vi "Main.vi"(8 "error in":errorcluster, 11 "Check all Worker Queues in":refnum<class "_Check all Worker Queues.lvclass">) -> (0 "error out":errorcluster, 3 "Check all Worker Queues out":refnum<class "_Check all Worker Queues.lvclass">)   [LabVIEW 2017, in "_Check all Worker Queues.lvclass"]
doc: "The <b>Queued Message Handler</b> of the Worker that owns this VI."
uses:
  _Check all Worker Queues.lvclass
  C:/Program Files (x86)/National Instruments/LabVIEW 2017/vi.lib/addons/_Workers/Library/Classes/Worker/Worker.lvclass
  Initialization Data.ctl
  Response Cases.ctl
  <vilib>/addons/_Workers/Library/Case Label.ctl
  _Check all Worker Queues.lvclass/_Check all Worker Queues.ctl
  rwr_Get Number of Elements in all Queues.ctl
  rwr_Get Number of Elements in all Queues Reply.ctl
  <vilib>/addons/_Workers/Library/Classes/Message Queue/Message Queue.lvclass
  <vilib>/addons/_Workers/Library/Workers.lvlib
panel:
  out "Multicolumn Listbox":i32(listbox)
  in  "Check Queues":bool
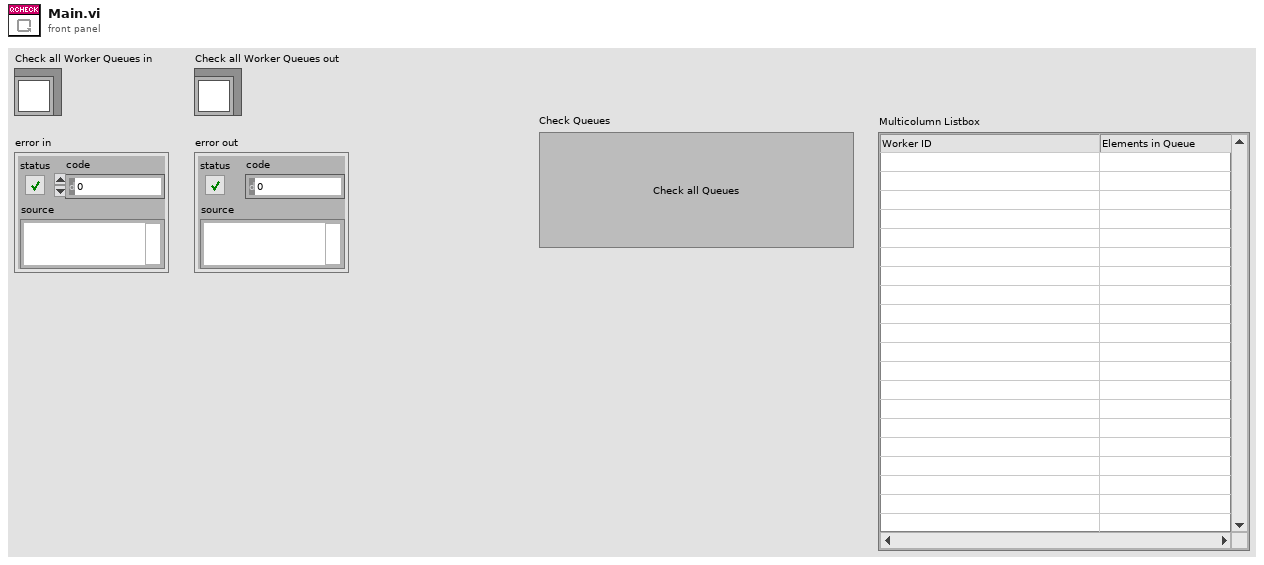
[diagram p1: front panel]
types:
  T1 = typedef "_Check all Worker Queues.lvclass/Initialization Data.ctl" = cluster{"Response Cases":T2}
  T2 = typedef "_Check all Worker Queues.lvclass/Response Cases.ctl" = cluster{"Placeholder - Can be deleted":string, "Get Number of Elements in all Queues_":T3}
  T3 = typedef "Workers.lvlib/Case Label.ctl" = string
  T4 = typedef "_Check all Worker Queues.lvclass/rwr_Get Number of Elements in all Queues Reply.ctl" = cluster{"Elements in Queues":string[][]}
  T5 = typedef "_Check all Worker Queues.lvclass/rwr_Get Number of Elements in all Queues.ctl" = cluster{"String":string}
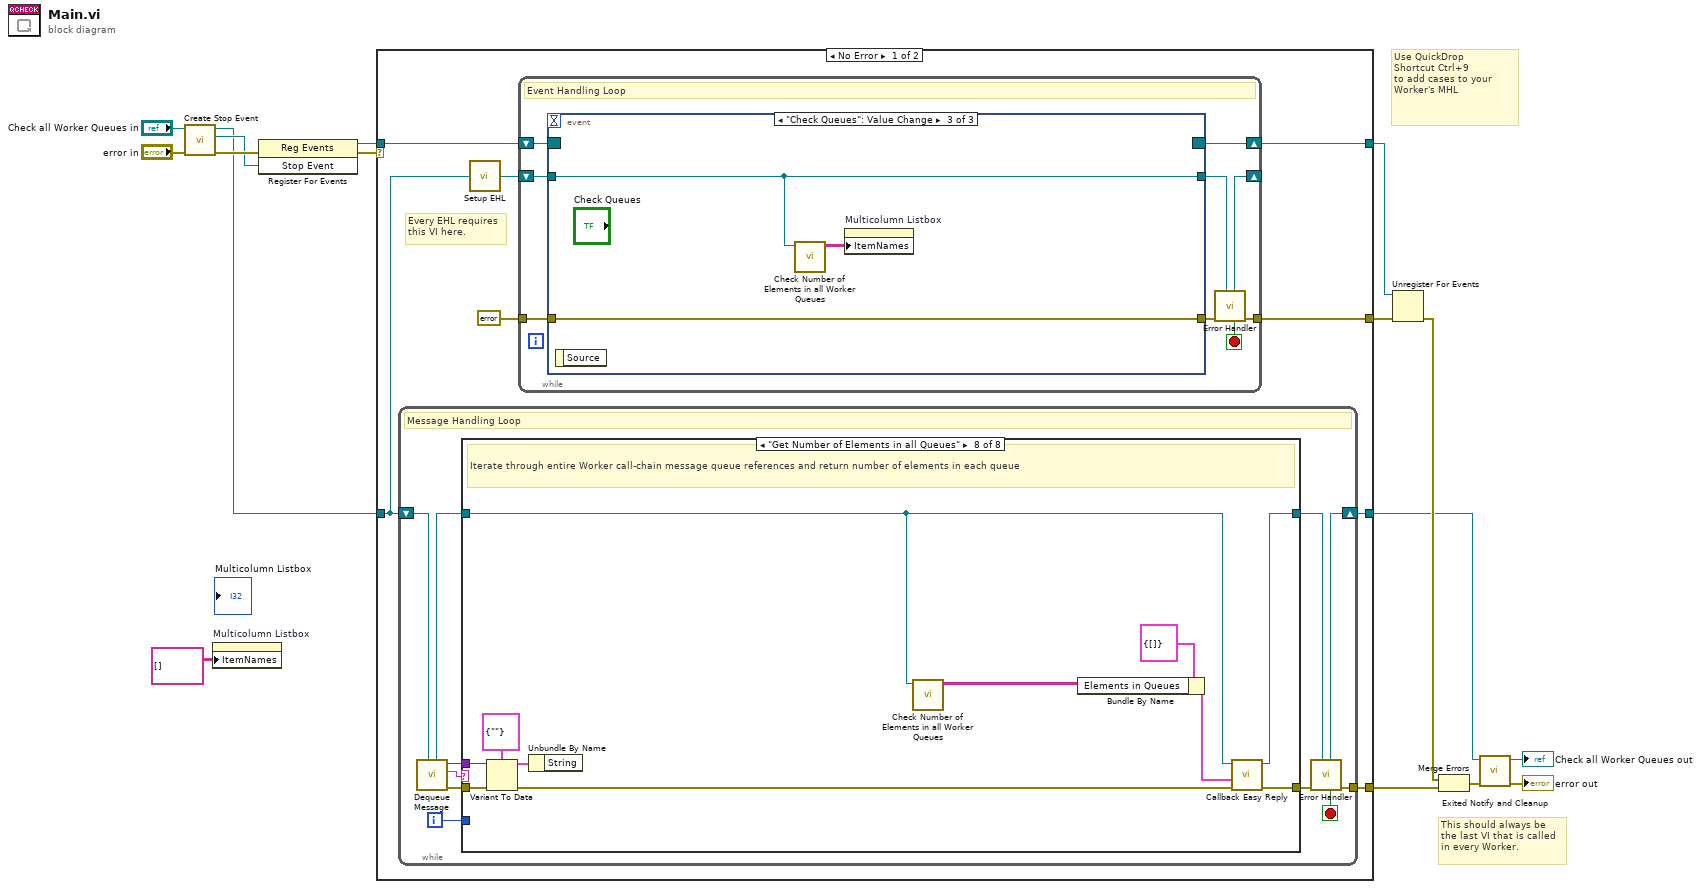
[diagram p0: block diagram]
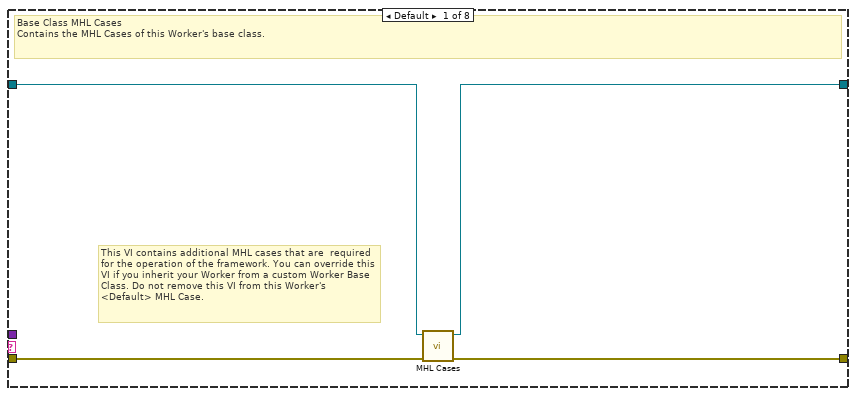
[diagram p2: hidden frame]
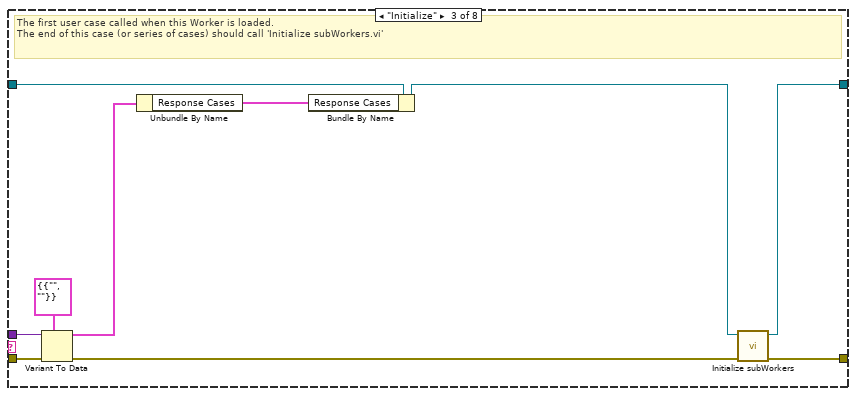
[diagram p4: hidden frame]
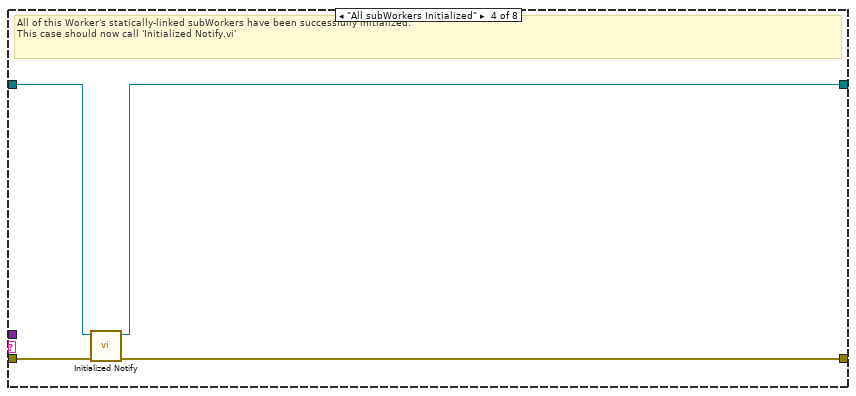
[diagram p5: hidden frame]
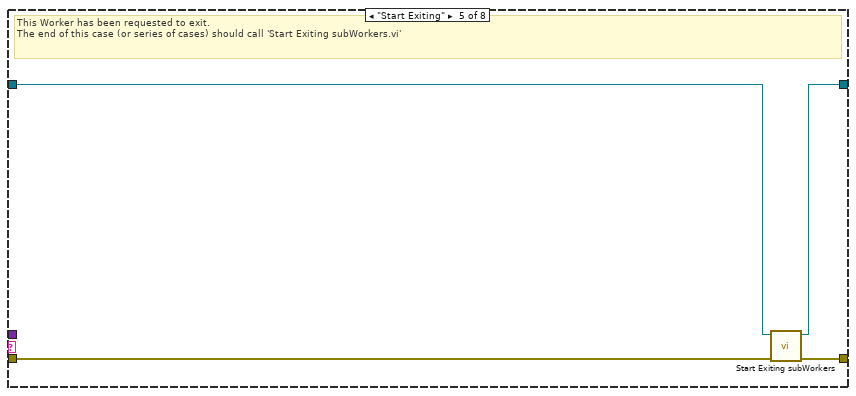
[diagram p6: hidden frame]
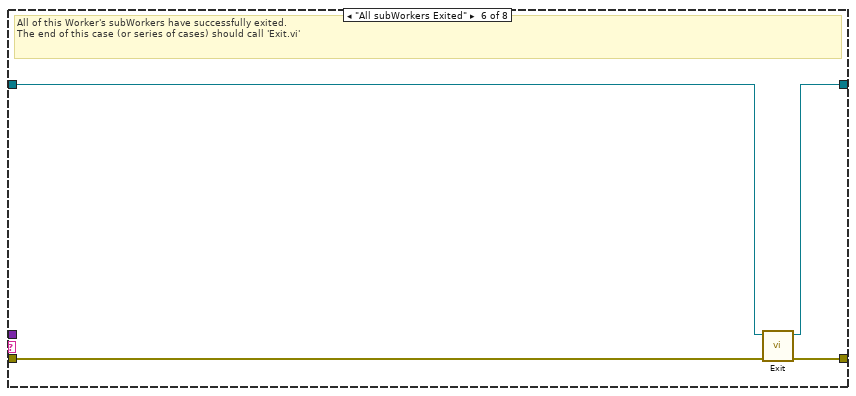
[diagram p7: hidden frame]
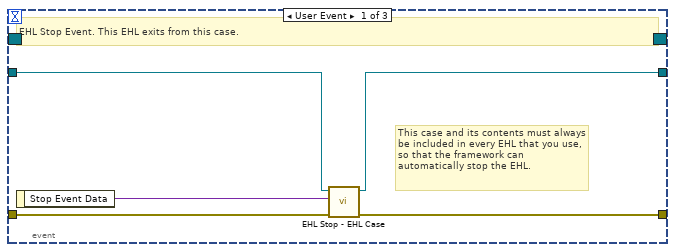
[diagram p9: hidden frame]
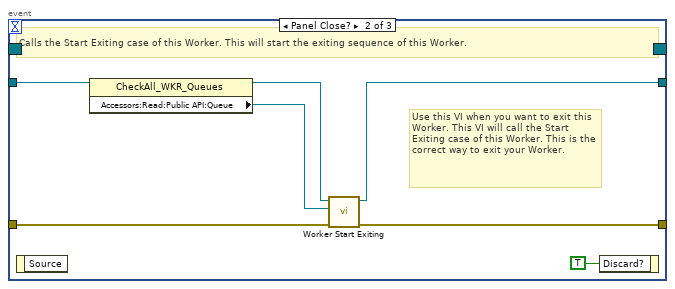
[diagram p10: hidden frame]
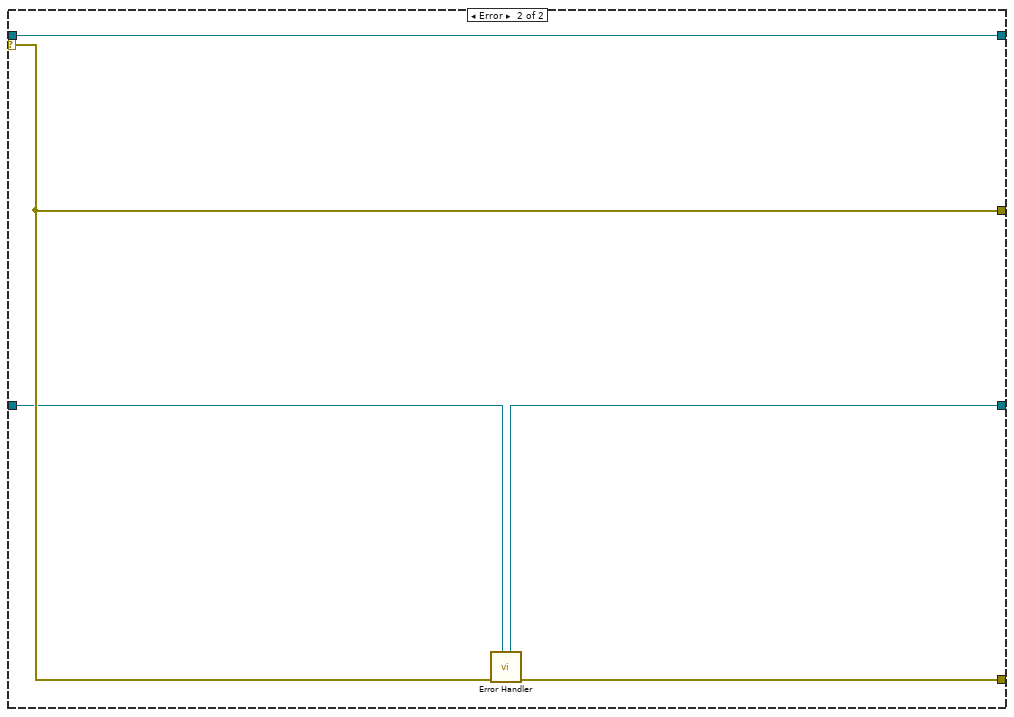
[diagram p11: hidden frame]
diagram:
  # "Use QuickDrop\nShortcut Ctrl+9\nto add cases to your\nWorker's MHL"
  # "This should always be the last VI that is called in every Worker."
  n1 = call-dynamic "Create Stop Event.vi"("error in"="error in", "Worker"="Check all Worker Queues in") -> ("error out"=w11:errorcluster, "Stop Event"=w8:refnum<user-event>, "Worker out"=w5:refnum<class "_Check all Worker Queues.lvclass">)  [unwired: 7 in]
  n2 = property on="Multicolumn Listbox" class="MCListbox (strict)"("ItemNames"=string[][] [] ("Item Names")) -> ()  [unwired: 2 in, 2 out]
  n3 = register-events(error in=w11, w8) -> (reference out=w10:refnum<event-registration>, error out=w2:errorcluster)  [unwired: 1 in]
  n4 = case shown="No Error" w2 {
    tunnel: w5 -> [w19 w102]
    tunnel: [w17 w103] -> w9
    tunnel: w10 -> [w24 w104]
    tunnel: [w21 w105] -> w15
    tunnel: [w23 w104] -> w14
    tunnel: [w18 w101] -> w12
    selector: w2 -> [_ w105]
    frame No Error {
      # "Every EHL requires\nthis VI here."
      n5 = while {
        shift-right: [w33] -> w18
        shift-left: w19 -> [w35]
        tunnel: [w34] -> w17
        i -> [w26]
        stop <- w27 stop-if-true
        # "Message Handling Loop"
        n6 = call-dynamic "Dequeue Message.vi"("Worker"=w35) -> ("error out"=w32:errorcluster, "Case out"=w28:string, "Data out"=w25:variant, "Worker out"=w30:refnum<class "_Check all Worker Queues.lvclass">)  [unwired: 6 in, 1 out]
        n7 = case "Worker MHL Case Structure (DO NOT CHANGE LABEL NAME)" shown="\"Get Number of Elements in all Queues\"" w28 {
          tunnel: w32 -> [w39 w40 w49 w53 w56 w63 w65 w76]
          tunnel: [w38 w40 w51 w52 w59 w62 w65 w71] -> w31
          tunnel: w30 -> [w37 w41 w48 w55 w57 w61 w64 w68]
          tunnel: [w36 w41 w50 w54 w58 w60 w64 w70] -> w29
          tunnel: w26 -> [_ _ _ _ _ _ _ _]
          tunnel: w25 -> [_ _ w46 _ _ _ _ w73]
          frame Default {
            # "This VI contains additional MHL cases that are  required for the operation of the framework. You can override this VI if you inherit your Worker from a custom Worker Base Class. Do not remove this VI from this Worker's <Default> MHL Case."
            # "Base Class MHL Cases\nContains the MHL Cases of this Worker's base class."
            n8 = call-dynamic "MHL Cases.vi"("error in"=w39, "Worker in"=w37) -> ("error out"=w38:errorcluster, "Worker out"=w36:refnum<class "_Check all Worker Queues.lvclass">)  [unwired: 8 in]
          }
          frame "------------ FRAMEWORK CASES -----------" {
            # "Start of Workers Framework Cases"
          }
          frame "Initialize" {
            # "The first user case called when this Worker is loaded.\nThe end of this case (or series of cases) should call 'Initialize subWorkers.vi'"
            n9 = Variant To Data(error in=w49, type=T1 {"Response Cases"={"Placeholder - Can be deleted"="", "Get Number of Elements in all Queues_"=""}} ("Initialization Data"), Variant=w46) -> (data=w44:T1, error out=w47:errorcluster)
            n10 = Unbundle By Name(w44) -> ("Response Cases"=w43:T2)
            n11 = Bundle By Name(cluster=w48, "Response Cases"=w43) -> (w45:refnum<class "_Check all Worker Queues.lvclass">)
            n12 = call-dynamic "Initialize subWorkers.vi"("error in"=w47, "Worker"=w45) -> ("error out"=w51:errorcluster, "dup Worker out"=w50:refnum<class "_Check all Worker Queues.lvclass">)  [unwired: 8 in]
          }
          frame "All subWorkers Initialized" {
            # "All of this Worker's statically-linked subWorkers have been successfully initialized.\nThis case should now call 'Initialized Notify.vi'"
            n13 = call-dynamic "Initialized Notify.vi"("error in"=w53, "Worker"=w55) -> ("error out"=w52:errorcluster, "dup Worker out"=w54:refnum<class "_Check all Worker Queues.lvclass">)  [unwired: 8 in]
          }
          frame "Start Exiting" {
            # "This Worker has been requested to exit. \nThe end of this case (or series of cases) should call 'Start Exiting subWorkers.vi'"
            n14 = call-dynamic "Start Exiting subWorkers.vi"("error_in"=w56, "Worker"=w57) -> ("error out"=w59:errorcluster, "dup Worker out"=w58:refnum<class "_Check all Worker Queues.lvclass">)  [unwired: 8 in]
          }
          frame "All subWorkers Exited" {
            # "All of this Worker's subWorkers have successfully exited. \nThe end of this case (or series of cases) should call 'Exit.vi'"
            n15 = call-dynamic "Exit.vi"("error_in"=w63, "Worker"=w61) -> ("error out"=w62:errorcluster, "dup Worker out"=w60:refnum<class "_Check all Worker Queues.lvclass">)  [unwired: 8 in]
          }
          frame "------------- PUBLIC API CASES -------------" {
            # "Start of Workers Public API Cases"
          }
          frame "Get Number of Elements in all Queues" {
            # "Iterate through entire Worker call-chain message queue references and return number of elements in each queue"
            n16 = Variant To Data(error in=w76, type=T5 {"String"=""} ("Data"), Variant=w73) -> (data=w72:T5, error out=w75:errorcluster)
            n17 = Unbundle By Name(w72) -> ()  [unwired: 1 out]
            n18 = call "Check Number of Elements in all Worker Queues.vi"("CheckAll_WKR_Queues in"=w68) -> ("Array"=w66:string[][])  [unwired: 10 in]
            n19 = Bundle By Name(cluster=T4 {"Elements in Queues"=[]} ("Reply Data"), "Elements in Queues"=w66) -> (w67:T4)
            n20 = call-dynamic "Callback Easy Reply.vi"("error in"=w75, "Data"=w67, "Worker"=w68) -> ("error out"=w71:errorcluster, "dup Worker out"=w70:refnum<class "_Check all Worker Queues.lvclass">)  [unwired: 7 in]
          }
        }
        n21 = call-dynamic "Error Handler.vi"("Worker"=w29, "error_in"=w31) -> ("error out"=w34:errorcluster, "Stop Loop"=w27:bool, "Worker out"=w33:refnum<class "_Check all Worker Queues.lvclass">)  [unwired: 7 in]
      }
      n22 = call-dynamic "Setup EHL.vi"("Worker"=w19) -> ("Worker out"=w20:refnum<class "_Check all Worker Queues.lvclass">)  [unwired: 14 in]
      n23 = while "Event Handling Loop" {
        shift-right: [w85] -> w23
        shift-left: w24 -> [w84]
        tunnel: [w80] -> w21
        tunnel: errorcluster {"status"=FALSE, "code"=0, "source"=""} ("error constant") -> [w82]
        shift-right: [w78] -> _
        shift-left: w20 -> [w83]
        stop <- w77 stop-if-true
        # "Event Handling Loop"
        n24 = event shown="[2] \"Check Queues\": Value Change" {
          selector: w84 -> [_ _ _]
          dyn-events: [_ _ _] -> w85
          timeout: _ -> [_ _ _]
          tunnel: [w89 w96 w100] -> w81
          tunnel: w82 -> [w90 w95 w100]
          tunnel: w83 -> [w88 w94 w98]
          tunnel: [w87 w93 w98] -> w79
          event User Event {
            # "This case and its contents must always be included in every EHL that you use, so that the framework can automatically stop the EHL."
            # "EHL Stop Event. This EHL exits from this case."
            n25 = event-data() -> ("Stop Event Data"=w86:variant)  [unwired: 1 in]
            n26 = call-dynamic "EHL Stop - EHL Case.vi"("error in"=w90, "Stop Event Data"=w86, "Worker"=w88) -> ("error out"=w89:errorcluster, "Worker out"=w87:refnum<class "_Check all Worker Queues.lvclass">)  [unwired: 7 in]
          }
          event Panel Close? {
            # "Use this VI when you want to exit this Worker. This VI will call the Start Exiting case of this Worker. This is the correct way to exit your Worker."
            # "Calls the Start Exiting case of this Worker. This will start the exiting sequence of this Worker."
            n27 = event-data() -> ()  [unwired: 1 in, 1 out]
            n28 = property class="CheckAll_WKR_Queues"(reference=w94) -> (reference out=w92:refnum<class "_Check all Worker Queues.lvclass">, "Accessors:Read:Public API:Queue"=w91:refnum<class "Message Queue.lvclass">)  [unwired: 1 in, 1 out]
            n29 = call-dynamic "Worker Start Exiting.vi"("error_in"=w95, "Message Queue"=w91, "Worker"=w92) -> ("error out"=w96:errorcluster, "dup Worker out"=w93:refnum<class "_Check all Worker Queues.lvclass">)  [unwired: 7 in]
            n30 = event-data("Discard?"=TRUE) -> ()  [unwired: 1 in, 1 out]
          }
          event "Check Queues": Value Change {
            n31 = event-data() -> ()  [unwired: 1 in, 1 out]
            n32 = call "Check Number of Elements in all Worker Queues.vi"("CheckAll_WKR_Queues in"=w98) -> ("Array"=w99:string[][])  [unwired: 10 in]
            n33 = property on="Multicolumn Listbox" class="MCListbox (strict)"("ItemNames"=w99) -> ()  [unwired: 2 in, 2 out]
          }
        }
        n34 = call-dynamic "Error Handler.vi"("Worker"=w79, "error_in"=w81) -> ("error out"=w80:errorcluster, "Stop Loop"=w77:bool, "Worker out"=w78:refnum<class "_Check all Worker Queues.lvclass">)  [unwired: 7 in]
      }
    }
    frame Error {
      n35 = call-dynamic "Error Handler.vi"("Worker"=w102, "error_in"=w105) -> ("error out"=w103:errorcluster, "Worker out"=w101:refnum<class "_Check all Worker Queues.lvclass">)  [unwired: 7 in, 1 out]
    }
  }
  n36 = Unregister For Events(event registration refnum=w14, error in=w15) -> (error out=w16:errorcluster)
  n37 = Merge Errors(w16, w9) -> (w13:errorcluster)
  n38 = call-dynamic "Exited Notify and Cleanup.vi"("error_in"=w13, "Worker"=w12) -> ("error out"=→"error out":errorcluster, "dup Worker out"=→"Check all Worker Queues out":refnum<class "_Check all Worker Queues.lvclass">)  [unwired: 8 in]
